vi "Get Optimiser Cell.vi"(8 "error in (no error)":errorcluster, 11 "Optimiser SBlock in":refnum<class "Optimiser SBlock.lvclass">) -> (0 "error out":errorcluster, 2 "Optimiser Cell":refnum<class "Optimiser Cell.lvclass">, 3 "Optimiser SBlock out":refnum<class "Optimiser SBlock.lvclass">)   [LabVIEW 2020, in "Run Utilities.lvlib" / "Optimiser SBlock.lvclass"]
uses:
  Optimiser SBlock.lvclass
  C:/Users/marco/Documents/GitHub_Lab/TALOS/talos/Run Utilities/Schedule Block/Schedule Block.lvclass
  Optimiser Cell/Optimiser Cell.lvclass
  Ancestor/Ancestor/Ancestor.lvclass/Ancestor.ctl
  Support VIs/Generate Error.vi
  FGV/Error Memory/Get Error Description.vi
  Support VIs/Get PC name.vi
  Ancestor/Ancestor/Read ID.vi
  Support VIs/Get Class Name.vi
  <vilib>/Utility/error.llb/Clear Errors.vi
  FGV/Error Memory/Error Memory Core.vi
  <vilib>/AdvancedString/Delimited String to 1D String Array.vi
  Support VIs/Circus Root Path.vi
  FGV/Error Memory/Error Crt Lvl checker.vi
  FGV/Error Memory/Error Memory Core.vi/40c8088d-b597-4017-91af-faa98e00292e.vi
  FGV/Error Memory/Error Memory Core.vi/d4a3ab98-063c-4e44-b43d-fbdcfe6c2be2.vi
  Support VIs/Global Memory.vi
  <vilib>/Utility/LVClass/Get LV Class Name.vi
  Support VIs/Is in Packed Library.vi
  Support VIs/TALOS Root path.vi
  Support VIs/Read CSV worksheet.vi
  Support VIs/Global Constants.vi
  <vilib>/Utility/error.llb/General Error Handler.vi
  Support VIs/Error Log.vi
  Schedule/Schedule.lvclass
  Ancestor/Ancestor/Ancestor.lvclass
  <vilib>/Comparison/Equal/Equal Functor/Equal Functor.lvclass
  TALOS.lvlib
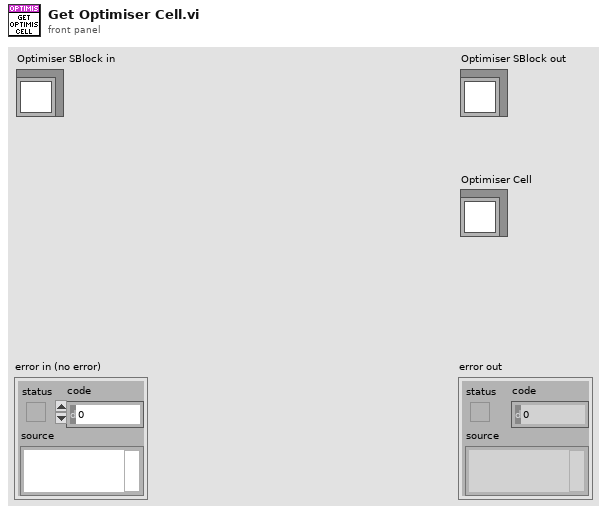
[diagram p1: front panel]
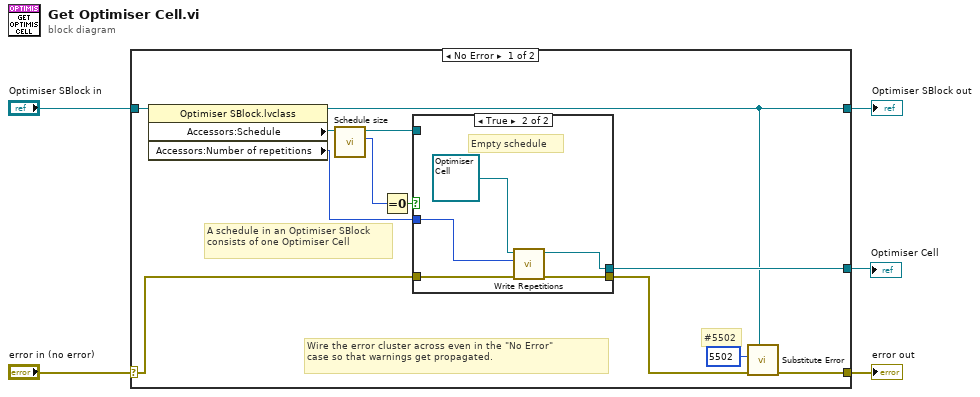
[diagram p0: block diagram]
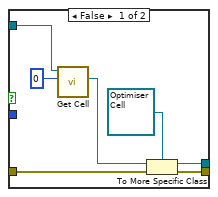
[diagram p2: hidden frame]
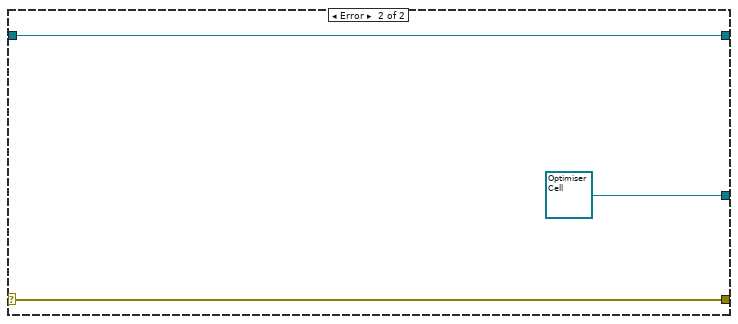
[diagram p3: hidden frame]
diagram:
  n1 = case shown="No Error" "error in (no error)" {
    selector: "error in (no error)" -> [w16 w32]
    tunnel: [w9 w32] -> w4
    tunnel: [w10 w31] -> w2
    tunnel: "Optimiser SBlock in" -> [w17 w31]
    tunnel: [w15 refnum<class "Optimiser Cell.lvclass"> refnum ("Scheduling.lvlib:Optimiser Cell.lvclass")] -> w1
    frame No Error {
      # "#5502"
      # "A schedule in an Optimiser SBlock consists of one Optimiser Cell"
      # "Wire the error cluster across even in the \"No Error\"\ncase so that warnings get propagated."
      n2 = property class="Optimiser SBlock.lvclass"(reference=w17) -> (reference out=w10:refnum<class "Optimiser SBlock.lvclass">, "Accessors:Schedule"=w14:refnum<class "Schedule.lvclass">, "Accessors:Number of repetitions"=w6:u16)  [unwired: 1 in, 1 out]
      n3 = call-dynamic "Schedule size.vi"("Schedule in"=w14) -> ("Size"=w13:i32, "Schedule out"=w11:refnum<class "Schedule.lvclass">)  [unwired: 8 in, 1 out]
      n4 = Equal To 0?(x=w13) -> (x = 0?=w12:bool)
      n5 = case shown="True" w12 {
        tunnel: w16 -> [w22 w29]
        tunnel: [w21 w28] -> w8
        tunnel: [w19 w27] -> w15
        tunnel: w11 -> [w18 _]
        tunnel: w6 -> [_ w25]
        frame False {
          n6 = call-dynamic "Get Cell.vi"("index"=0, "Schedule in"=w18) -> ("Schedule Cell"=w23:refnum<class "Schedule Cell.lvclass">)  [unwired: 7 in, 2 out]
          n7 = To More Specific Class(target class=refnum<class "Optimiser Cell.lvclass"> refnum ("Scheduling.lvlib:Optimiser Cell.lvclass"), reference=w23, error in=w22) -> (specific class reference=w19:refnum<class "Optimiser Cell.lvclass">, error out=w21:errorcluster)
        }
        frame True {
          # "Empty schedule"
          n8 = call-dynamic "Write Repetitions.vi"("error in (no error)"=w29, "Repetitions"=w25, "Schedule Cell in"=refnum<class "Optimiser Cell.lvclass"> refnum ("Scheduling.lvlib:Optimiser Cell.lvclass")) -> ("error out"=w28:errorcluster, "Schedule Cell out"=w27:refnum<class "Optimiser Cell.lvclass">)  [unwired: 7 in]
        }
      }
      n9 = call "Substitute Error.vi"("LabVIEW Object"=w10, "error in (no error)"=w8, "Error Code"=5502) -> ("error out"=w9:errorcluster)  [unwired: 8 in]
    }
    frame Error {
    }
  }
  "error out" <- w4
  "Optimiser SBlock out" <- w2
  "Optimiser Cell" <- w1
